vi "Player Info.vi"(11 "Coward in":refnum<class "Sir Robin.lvclass">) -> (0 "Defeat Speech":string, 1 "Victory Speech":string, 2 "Name":string, 3 "Coward out":refnum<class "Sir Robin.lvclass">)   [LabVIEW 2015, in "Sir Robin.lvclass"]
uses:
  Sir Robin.lvclass
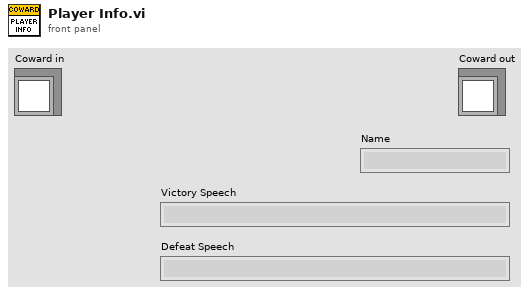
[diagram p1: front panel]
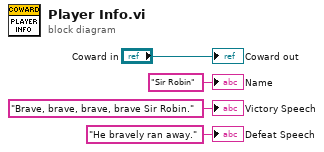
[diagram p0: block diagram]
diagram:
  "Coward out" <- "Coward in"
  "Name" <- "Sir Robin" ("Name")
  "Victory Speech" <- "Brave, brave, brave, brave Sir Robin." ("Victory Speech")
  "Defeat Speech" <- "He bravely ran away." ("Defeat Speech")
